vi "ma_concatenate waveforms (array).vi"(0 "Waveforms A0 in":waveform(dbl)[](array[waveform]), 5 "Waveforms A1 in":waveform(dbl)[](array[waveform]), 11 "error in":errorcluster) -> (4 "Waveforms A out":waveform(dbl)[](array[waveform]), 15 "error out":errorcluster)   [LabVIEW 2020, in "NI_MAPro.lvlib"]
uses:
  NI_MAPro.lvlib
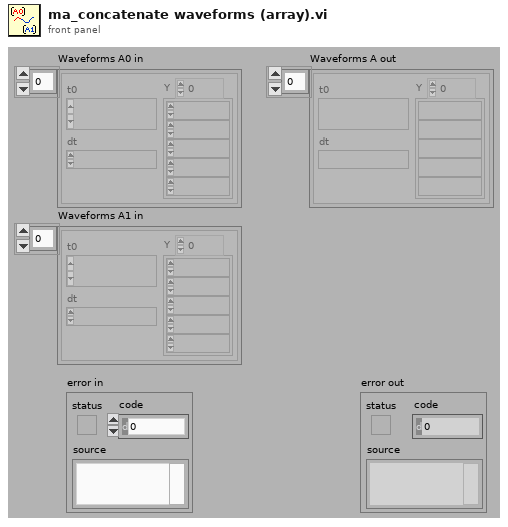
[diagram p1: front panel]
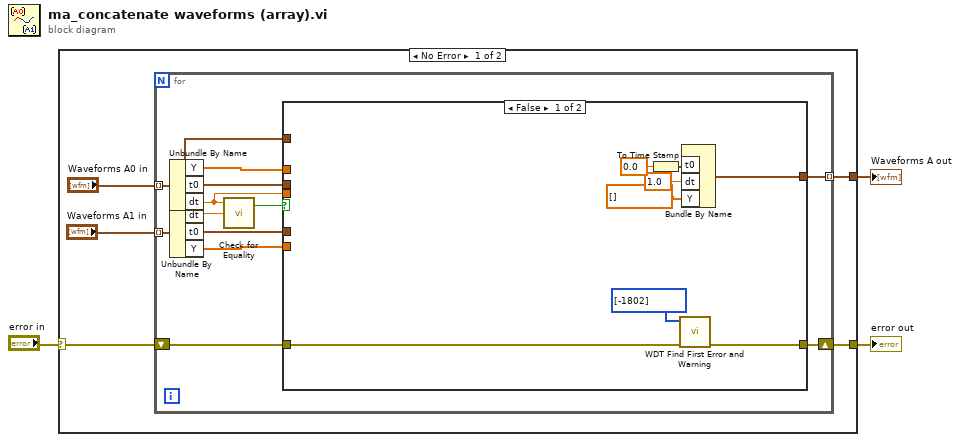
[diagram p0: block diagram]
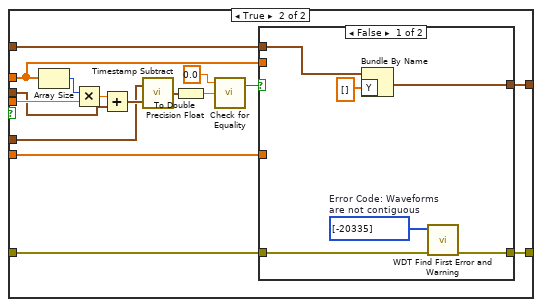
[diagram p2: hidden frame]
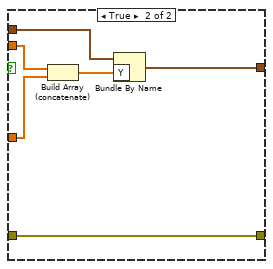
[diagram p3: hidden frame]
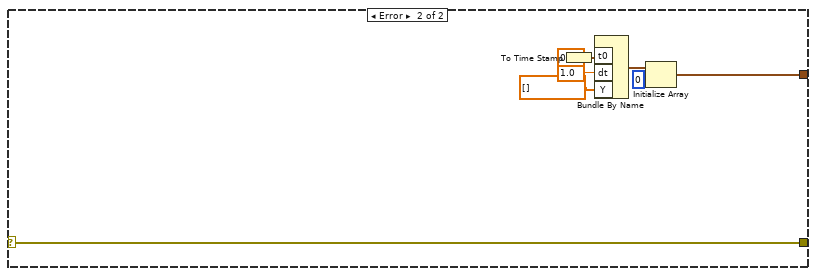
[diagram p4: hidden frame]
diagram:
  n1 = case shown="No Error" "error in" {
    selector: "error in" -> [w6 w64]
    tunnel: [w5 w64] -> w2
    tunnel: [w4 w58] -> w1
    frame No Error {
      n2 = for {
        tunnel: "Waveforms A0 in" -> [w15] mode=indexing
        tunnel: "Waveforms A1 in" -> [w14] mode=indexing
        shift-right: [w12] -> w5
        shift-left: w6 -> [w13]
        tunnel: [w11] -> w4 mode=indexing
        n3 = Unbundle By Name(w15) -> ("Y"=w18:dbl[], "t0"=w10:timestamp, "dt"=w17:dbl)
        n4 = Unbundle By Name(w14) -> ("dt"=w20:dbl, "t0"=w9:timestamp, "Y"=w16:dbl[])
        n5 = call "Check for Equality.vi"("n2"=w20, "n1"=w17) -> ("equal?"=w19:bool)  [unwired: 1 in, 1 out]
        n6 = case shown="False" w19 {
          tunnel: w13 -> [w28 w36]
          tunnel: w18 -> [_ w39]
          tunnel: w17 -> [_ w43]
          tunnel: w10 -> [_ w41]
          tunnel: w9 -> [_ w32]
          tunnel: w16 -> [_ w38]
          tunnel: w15 -> [_ w37]
          tunnel: [w26 w35] -> w12
          tunnel: [w25 w34] -> w11
          frame False {
            n7 = To Time Stamp(1:0.0 ("t0")) -> (0:w21:timestamp)
            n8 = call "WDT Find First Error and Warning.vi"("error in (no error)"=w28, "Error Codes"=i32[] [-1802]) -> ("error out"=w26:errorcluster)  [unwired: 4 in, 1 out]
            n9 = Bundle By Name("t0"=w21, "dt"=1.0, "Y"=dbl[] []) -> (w25:waveform(dbl))  [unwired: 1 in]
          }
          frame True {
            n10 = Array Size(array=w39) -> (size(s)=w44:i32)
            n11 = Multiply(x=w44, y=w43) -> (x*y=w42:dbl)
            n12 = Add(x=w42, y=w41) -> (x+y=w33:timestamp)
            n13 = call "Timestamp Subtract.vi"("y"=w33, "x"=w32) -> ("x - y"=w30:timestamp)
            n14 = To Double Precision Float(number=w30) -> (double precision float=w31:dbl)
            n15 = call "Check for Equality.vi"("n2"=w31, "n1"=0.0) -> ("equal?"=w40:bool)  [unwired: 1 in, 1 out]
            n16 = case shown="False" w40 {
              tunnel: w39 -> [_ w56]
              tunnel: w38 -> [_ w55]
              tunnel: w37 -> [w49 w53]
              tunnel: [w48 w52] -> w34
              tunnel: [w46 w51] -> w35
              tunnel: w36 -> [w47 w51]
              frame False {
                w45 = i32[] [-20335]  # Error Code: Waveforms are not contiguous
                n17 = Bundle By Name(cluster=w49, "Y"=dbl[] []) -> (w48:waveform(dbl))
                n18 = call "WDT Find First Error and Warning.vi"("error in (no error)"=w47, "Error Codes"=w45) -> ("error out"=w46:errorcluster)  [unwired: 4 in, 1 out]
              }
              frame True {
                n19 = Build Array (concatenate)(w56, w55) -> (w54:dbl[])
                n20 = Bundle By Name(cluster=w53, "Y"=w54) -> (w52:waveform(dbl))
              }
            }
          }
        }
      }
    }
    frame Error {
      n21 = To Time Stamp(1:0.0 ("t0")) -> (0:w57:timestamp)
      n22 = Bundle By Name("t0"=w57, "dt"=1.0, "Y"=dbl[] []) -> (w60:waveform(dbl))  [unwired: 1 in]
      n23 = Initialize Array(w60, 0 ("dimension size")) -> (w58:waveform(dbl)[])
    }
  }
  "error out" <- w2
  "Waveforms A out" <- w1
